vi "LinearSystemSim_SetInput_Single.vi"(8 "Battery_Volts":dbl=12.0, 9 "Input Value":dbl, 10 "Row":i32, 11 "in LinearSystemSim":T1) -> (3 "out LinearSystemSim":T1)   [LabVIEW 2019, in "Trajectory_Library.lvlib"]
doc: "Creates a new LINEAR SYSTEM data cluster with the specified values. \n\n\nInputs: \n - XXX -- XXX.\n\nOutputs:\n - XXX -- XXX."
uses:
  Trajectory_Library.lvlib
  LINEAR_SYSTEM_SIM.ctl
  LINEAR_SYSTEM.ctl
  <vilib>/Analysis/Matrix/Datatypes/RealMatrix.ctl
  <vilib>/Analysis/Matrix/NI_Matrix.lvlib
panel:
  # "<States, 1>"
  # "<Outputs, 1>"
  # "<Inputs, 1>"
  # "<Outputs, 1>"
  # "<States,States>"
  # "<States,Inputs>"
  # "<Outputs,States>"
  # "<Outputs,Inputs>"
  # "<States, 1>"
  # "<Outputs, 1>"
  # "<Inputs, 1>"
  # "<Outputs, 1>"
  # "<States,States>"
  # "<States,Inputs>"
  # "<Outputs,States>"
  # "<Outputs,Inputs>"
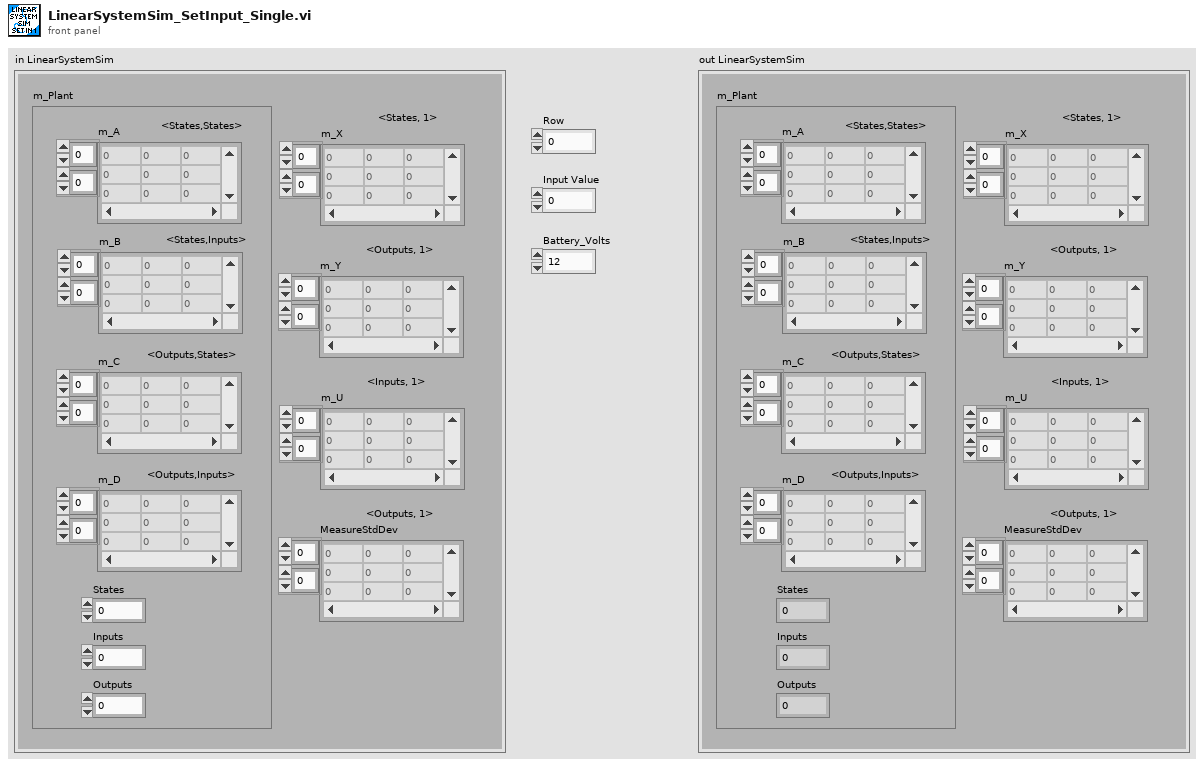
[diagram p1: front panel]
types:
  T1 = typedef "Trajectory_Library.lvlib/LINEAR_SYSTEM_SIM.ctl" = cluster{"m_Plant":T2, "m_X":T3, "m_Y":T3, "m_U":T3, "MeasureStdDev":T3}
  T2 = typedef "Trajectory_Library.lvlib/LINEAR_SYSTEM.ctl" = cluster{"m_A":T3, "m_B":T3, "m_C":T3, "m_D":T3, "States":i32, "Inputs":i32, "Outputs":i32}
  T3 = typedef "NI_Matrix.lvlib/RealMatrix.ctl" = dbl[][]
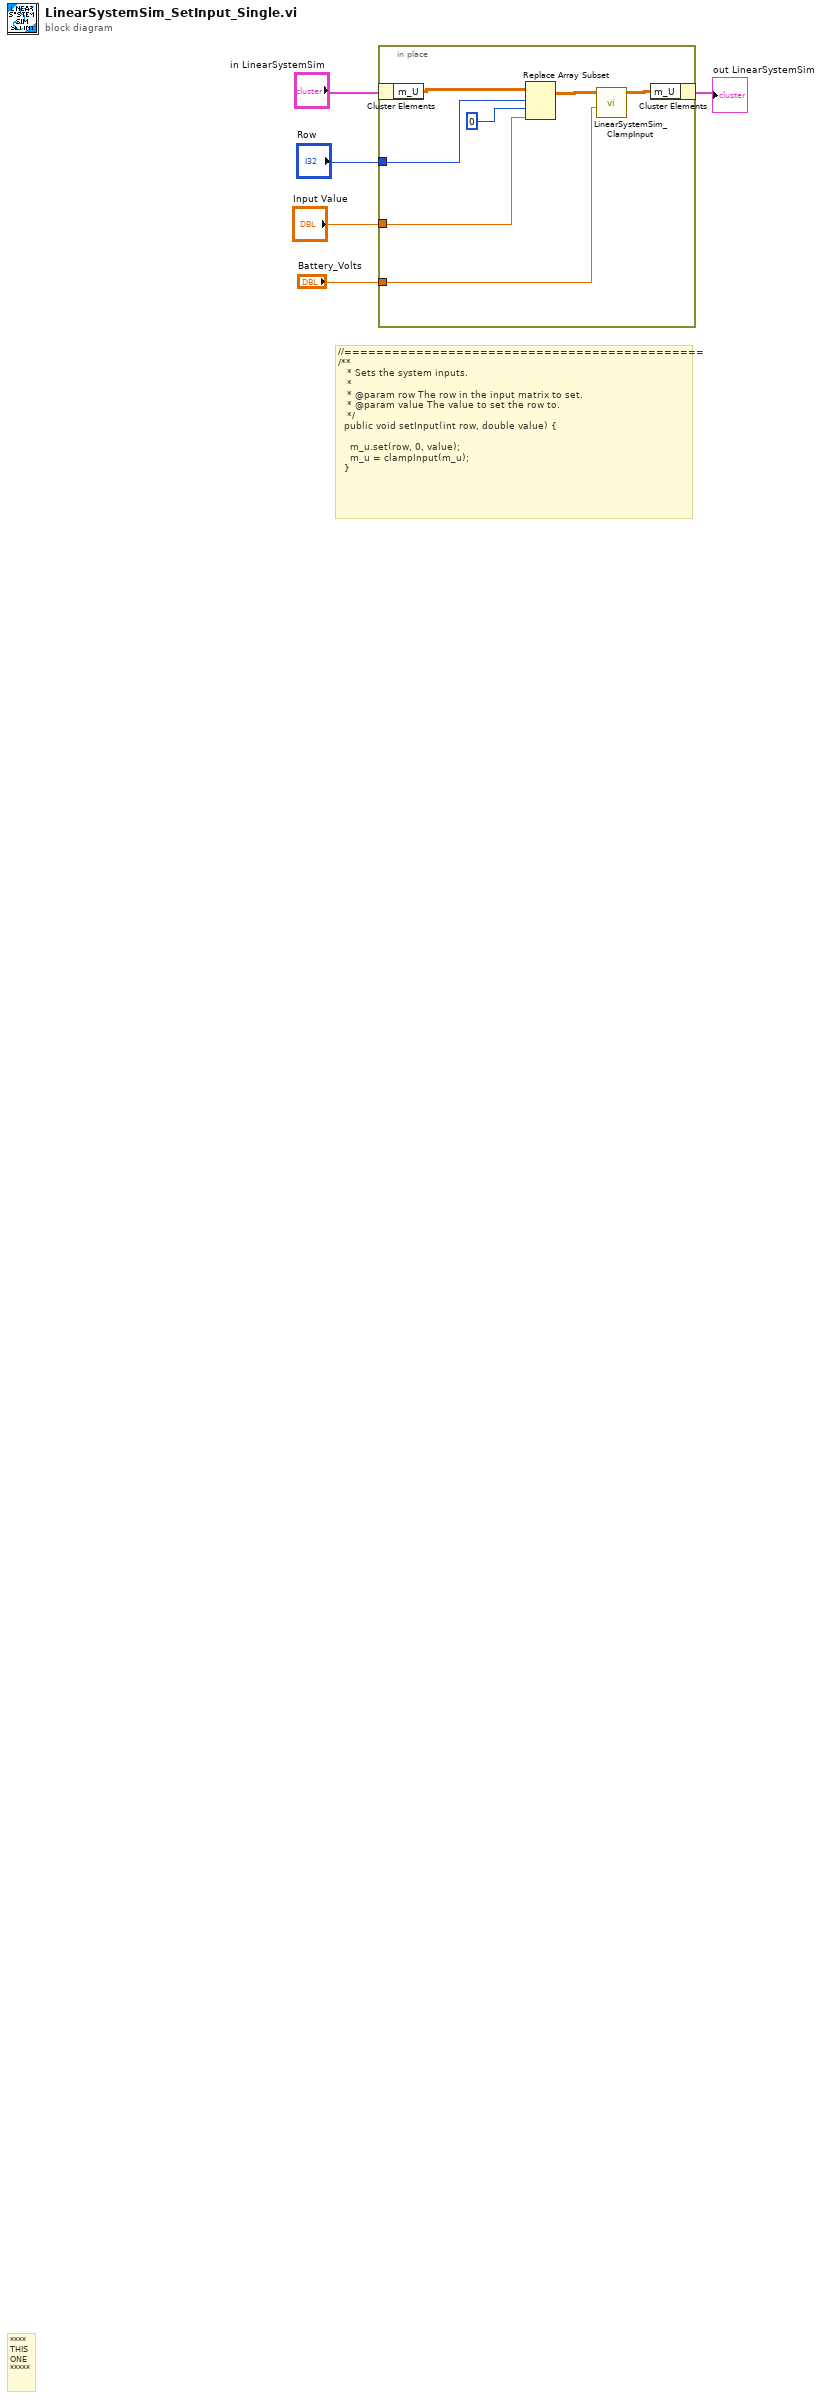
[diagram p0: block diagram]
diagram:
  # "//=============================================\n/**\n   * Sets the system inputs.\n   *\n   * @param row The row in the input matrix to set.\n   * @param value The value to set the row to.\n   */\n  public void setInput(int row, double value) {\n\n    m_u.set(row, 0, value);\n    m_u = clampInput(m_u);\n  }"
  # "****\nTHIS\nONE\n*****"
  n1 = in-place {
    in-place-border: "Input Value" -> [w9]
    in-place-border: "Row" -> [w11]
    in-place-border: "Battery_Volts" -> [w6]
    n2 = in-place-cluster #1("in LinearSystemSim") -> ("m_U"=w12:T3)
    n3 = Replace Array Subset(array=w12, new element=w9, index (row)=w11, index (col)=0 ("disabled index (col)")) -> (w7:T3)
    n4 = call "LinearSystemSim_ClampInput.vi"("Battery_Volts"=w6, "Input"=w7) -> ("ClampedInput"=w8:T3)  [unwired: 9 in]
    n5 = in-place-cluster #1("m_U"=w8) -> (→"out LinearSystemSim":T1)
  }
